vi "Stop Core.vi"(10 "final error code":i32, 11 "User Interface in":refnum<class "User Interface.lvclass">) -> (3 "User Interface out":refnum<class "User Interface.lvclass">)   [LabVIEW 2015, in "User Interface.lvlib" / "User Interface.lvclass"]
doc: "(<B>Filename</B>: Actor Framework.lvlib:Actor.lvclass:Stop Core.vi)\n\nDefines what the actor does before it stops. Use the <B>final error code</B> input to determine whether the actor shut down in response to an error.\n\nBy default, this method does nothing. A descendant class may override it to define behavior, such as shutting down any processes the actor initiated in its override of the Actor Core method."
uses:
  User Interface.lvclass
  User Interface.lvclass/User Interface.ctl
  <vilib>/ActorFramework/Actor/Actor.lvclass
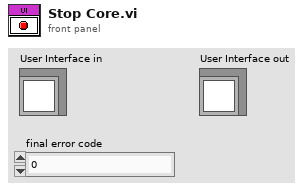
[diagram p1: front panel]
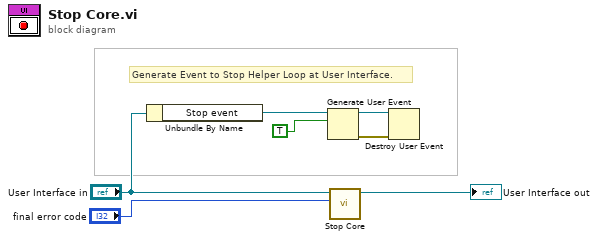
[diagram p0: block diagram]
diagram:
  # "Generate Event to Stop Helper Loop at User Interface."
  n1 = Unbundle By Name("User Interface in") -> ("Stop event"=w4:refnum<user-event>)
  n2 = Generate User Event(user event=w4, event data cluster=TRUE) -> (user event out=w2:refnum<user-event>, error out=w1:errorcluster)  [unwired: 2 in]
  n3 = call-parent "Stop Core.vi"("final error code"="final error code", "Actor in"="User Interface in") -> ("Actor out"=→"User Interface out":refnum<class "User Interface.lvclass">)  [unwired: 9 in]
  n4 = Destroy User Event(user event=w2, error in=w1) -> ()  [unwired: 1 out]
